vi "Teach Click Position.vi"(2 "Wait time (s)":i32=5, 3 "Click position file path":path) -> (0 "Y":i32, 1 "X":i32)   [LabVIEW 2015]
panel:
  out "Error out":errorcluster
  out "Time remaining (s)":i32
  # "PN 18/11/2015"
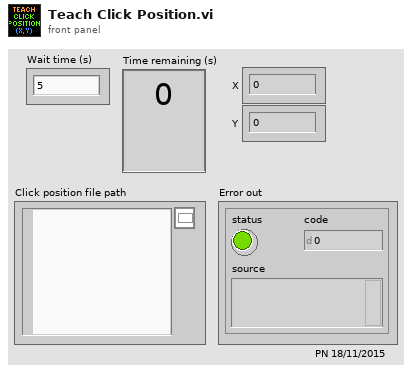
[diagram p1: front panel]
types:
  T1 = enum16{"open", "replace", "create", "open or create", "replace or create", "replace or create with confirmation"}
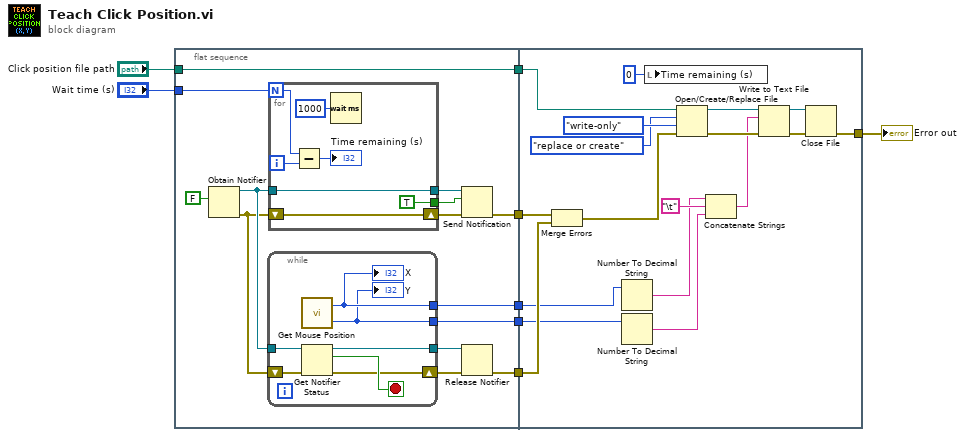
[diagram p0: block diagram]
diagram:
  n1 = flat-sequence {
    tunnel: "Wait time (s)" -> [w22]
    tunnel: [w13] -> w7
    tunnel: [w12] -> w6
    tunnel: [w11] -> w5
    tunnel: [w10] -> w4
    tunnel: [w9] -> w2
    tunnel: "Click position file path" -> [w9]
    tunnel: w7 -> [w44]
    tunnel: w6 -> [w45]
    tunnel: w5 -> [w50]
    tunnel: w4 -> [w49]
    tunnel: [w38] -> w3
    tunnel: w2 -> [w37]
    frame #0 {
      n2 = Obtain Notifier(notification data type=FALSE) -> (notifier out=w19:refnum<notifier>, error out=w15:errorcluster)  [unwired: 3 in, 1 out]
      n3 = while {
        tunnel: [w24] -> w13
        tunnel: [w23] -> w12
        tunnel: [w28] -> w20
        tunnel: w19 -> [w27]
        shift-right: [w25] -> w14
        shift-left: w15 -> [w26]
        stop <- w29 stop-if-true
        n4 = call "Get Mouse Position.vi"() -> ("X"=w24:i32, "Y"=w23:i32)  [unwired: 1 in]
        "X" <- w24
        "Y" <- w23
        n5 = Get Notifier Status(notifier=w27, error in (no error)=w26) -> (notifier out=w28:refnum<notifier>, current notification=w29:bool, error out=w25:errorcluster)  [unwired: 2 out]
      }
      n6 = for {
        N: w22 -> [w35]
        tunnel: [TRUE] -> w17
        tunnel: w19 -> [w31]
        tunnel: [w31] -> w18
        shift-right: [w30] -> w16
        shift-left: w15 -> [w30]
        i -> [w34]
        n7 = Subtract(x=w35, y=w34) -> (x-y=→"Time remaining (s)":i32)
        n8 = Wait (ms)(milliseconds to wait=u32 1000) -> ()  [unwired: 1 out]
      }
      n9 = Send Notification(notification=w17, notifier=w18, error in (no error)=w16) -> (error out=w10:errorcluster)  [unwired: 1 out]
      n10 = Release Notifier(notifier=w20, error in (no error)=w14) -> (error out=w11:errorcluster)  [unwired: 1 in, 2 out]
    }
    frame #1 {
      n11 = Merge Errors(w49, w50) -> (w48:errorcluster)
      n12 = Number To Decimal String(number=w44) -> (decimal integer string=w43:string)  [unwired: 1 in]
      n13 = Number To Decimal String(number=w45) -> (decimal integer string=w42:string)  [unwired: 1 in]
      n14 = local write "Time remaining (s)"(0 ("Time remaining (s)")) -> ()
      n15 = Open/Create/Replace File(file path (use dialog)=w37, error in=w48, operation (0:open)=T1."replace or create", access (0:read/write)=enum16{"read/write", "read-only", "write-only"}."write-only") -> (refnum out=w47:refnum<file>, error out=w53:errorcluster)  [unwired: 2 in, 1 out]
      n16 = Concatenate Strings(w43, "\t", w42) -> (w41:string)
      n17 = Write to Text File(file (use dialog)=w47, text=w41, error in=w53) -> (refnum out=w39:refnum<file>, error out=w40:errorcluster)  [unwired: 1 in, 1 out]
      n18 = Close File(refnum=w39, error in=w40) -> (error out=w38:errorcluster)  [unwired: 1 out]
    }
  }
  "Error out" <- w3
